vi "BrowseTargetIPs.vi"(5 "error in (no error)":errorcluster) -> (14 "target IPs":string[](array[string]), 15 "target names":string[](array[string]), 16 "no targets?":bool, 19 "error out":errorcluster)   [LabVIEW 2017, in "G#RemoteProxy.lvclass"]
uses:
  <vilib>/addons/_AddQ/G#Debugger/G#RemoteProxy/G#RemoteProxy.lvclass
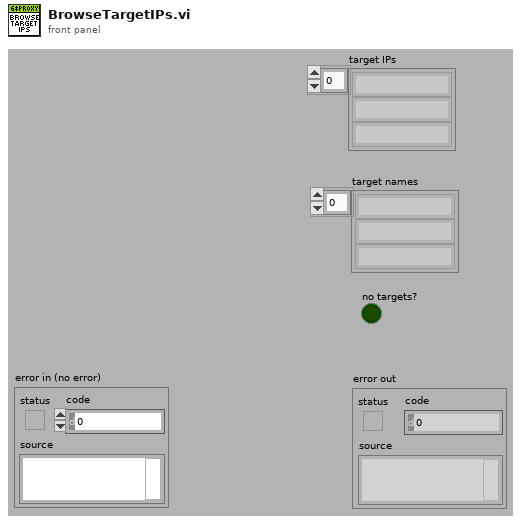
[diagram p1: front panel]
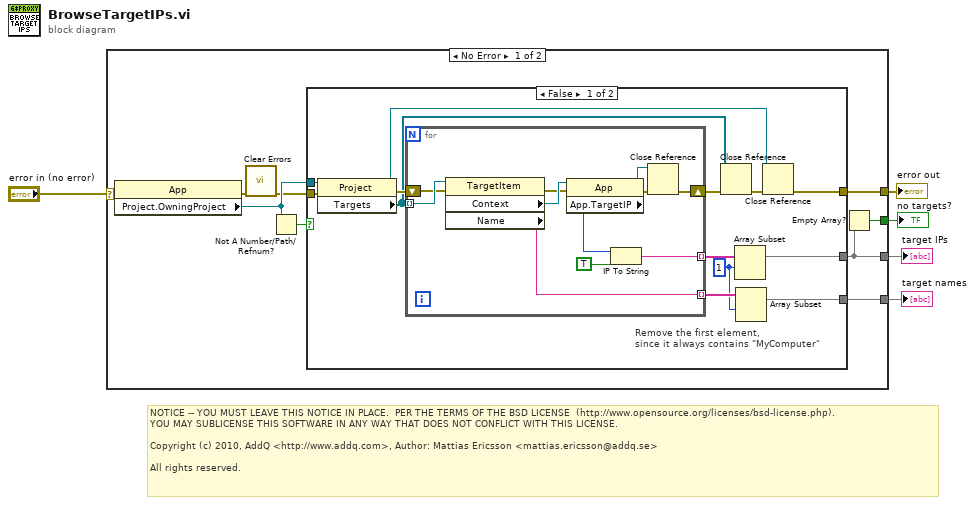
[diagram p0: block diagram]
diagram:
  # "NOTICE -- YOU MUST LEAVE THIS NOTICE IN PLACE.  PER THE TERMS OF THE BSD LICENSE  (http://www.opensource.org/licenses/bsd-license.php).\nYOU MAY SUBLICENSE THIS SOFTWARE IN ANY WAY THAT DOES NOT CONFLICT WITH THIS LICENSE.\n\nCopyright (c) 2010, AddQ <http://www.addq.com>, Author: Mattias Ericsson <mattias.ericsson@addq.se>\n\nAll rights reserved."
  n1 = case shown="No Error" "error in (no error)" {
    selector: "error in (no error)" -> [w8 w40]
    tunnel: [w10 w40] -> w5
    tunnel: [w7 _] -> w4
    tunnel: [w9 _] -> w3
    tunnel: [w6 _] -> w1
    frame No Error {
      n2 = property class="App"(error in=w8) -> (error out=w13:errorcluster, "Project.OwningProject"=w14:refnum<vi>)  [unwired: 1 in, 1 out]
      n3 = call <vilib>:"Clear Errors.vi"("error in (no error)"=w13) -> ("error out"=w12:errorcluster)  [unwired: 5 in, 1 out]
      n4 = Not A Number/Path/Refnum?(number/path/refnum=w14) -> (NaN/Path/Refnum?=w11:bool)
      n5 = case shown="False" w11 {
        tunnel: w14 -> [w27 _]
        tunnel: w12 -> [w25 w39]
        tunnel: [w20 w39] -> w10
        tunnel: [w18 _] -> w7
        tunnel: [w16 _] -> w9
        frame False {
          w15 = 1 ("index")
          # "Remove the first element,\nsince it always contains \"MyComputer\""
          n6 = property class="Project"(reference=w27, error in=w25) -> (reference out=w21:refnum<vi>, error out=w26:errorcluster, "Targets"=w23:refnum<vi>[])
          n7 = for {
            tunnel: w23 -> [w38] mode=indexing
            tunnel: [w35] -> w19 mode=indexing
            tunnel: [w33] -> w17 mode=indexing
            shift-right: [w28] -> w24
            shift-left: w26 -> [w32]
            n8 = property class="TargetItem"(reference=w38, error in=w32) -> (error out=w31:errorcluster, "Context"=w37:refnum<vi>, "Name"=w33:string)  [unwired: 1 out]
            n9 = property class="App"(reference=w37, error in=w31) -> (reference out=w29:refnum<vi>, error out=w30:errorcluster, "App.TargetIP"=w36:u32)
            n10 = IP To String(1:TRUE ("dot notation? (F)"), 2:w36) -> (0:w35:string)
            n11 = Close Reference(reference=w29, error in (no error)=w30) -> (error out=w28:errorcluster)
          }
          n12 = Close Reference(reference=w23, error in (no error)=w24) -> (error out=w22:errorcluster)
          n13 = Array Subset(array=w19, index=w15) -> (w18:string[])  [unwired: 1 in]
          n14 = Array Subset(array=w17, index=w15) -> (w16:string[])  [unwired: 1 in]
          n15 = Close Reference(reference=w21, error in (no error)=w22) -> (error out=w20:errorcluster)
        }
        frame True {
        }
      }
      n16 = Empty Array?(array=w7) -> (empty?=w6:bool)
    }
    frame Error {
    }
  }
  "error out" <- w5
  "target IPs" <- w4
  "target names" <- w3
  "no targets?" <- w1
